vi "Main_Module.vi"(0 "Instances":string(tree)="Addition_8", 11 "Error_In":errorcluster) -> (15 "Error_Out":errorcluster)   [LabVIEW 2021]
doc: "This is the main module that performs the calculator operation"
uses:
  Controls/Queue_Operation_Select.ctl
  Drivers/QD_Main.vi
  Controls/State_and_Data.ctl
  Classes/Calculator/Calculator.lvclass
  <vilib>/Utility/miscctls.llb/LVMapReplaceAction.ctl
  Controls/Object_Data.ctl
  Controls/Object_and_instance.ctl
  Controls/INI_Operation_Select.ctl
  Controls/Main_Module_Data.ctl
  Drivers/QD_Calci.vi
panel:
  in  "Load":bool
  in  "Save":bool
  in  "Delete":bool
  in  "Add":bool
  in  "Math_Functions":T1(ring) caption="Math Functions"
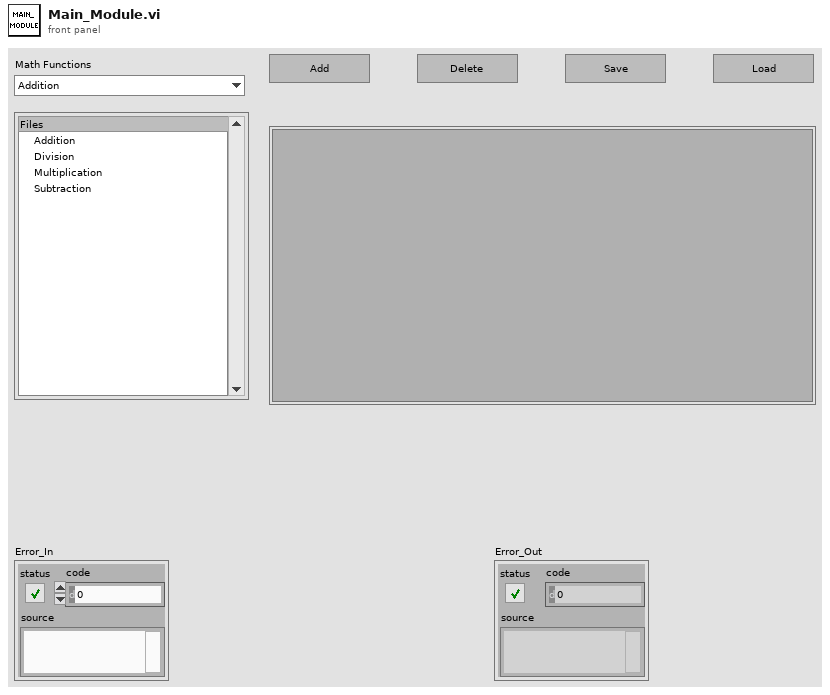
[diagram p1: front panel]
types:
  T1 = enum32{"Addition", "Division", "Multiplication", "Subtraction"}
  T2 = typedef "Queue_Operation_Select.ctl" = enum16{"Obtain_Queue", "Enqueue", "Enqueue_First", "Enqueue_N", "Lossy_Enqueue", "Preview", "Queue_Status", "Dequeue", "Flush", "Release_Queue"}
  T3 = typedef "Main_Module_Data.ctl" = cluster{"File_hierarchy_Reference":refnum<vi>, "Math_Function_Selected":string, "State_and_Data":T4, "Math_Functions":enum16{"Addition", "Division", "Multiplication", "Subtraction"}, "Parent_Class_Path":path, "Calculator.lvclass":refnum<class "Calculator.lvclass">, "Object_Data":T5, "Selected_Tag":string, "Calculator_File_Path":path, "Loaded_VI_Reference":refnum<vi>, "Loaded_Math_Function":string, "Loaded_Tag":string, "Total_Classes":string[], "INI_File_Path":path}
  T4 = typedef "State_and_Data.ctl" = cluster{"State":string, "Data":variant}
  T5 = typedef "Object_Data.ctl" = map{string, map{string, refnum<class "Calculator.lvclass">}}
  T6 = enum16{"Addition", "Division", "Multiplication", "Subtraction"}
  T7 = typedef "Object_and_instance.ctl" = cluster{"Object":refnum<class "Calculator.lvclass">, "Instance":string}
  T8 = typedef "INI_Operation_Select.ctl" = enum16{"Initialize", "Read", "Read_Key", "Write"}
  T9 = typedef "LVMapReplaceAction.ctl" = enum32{"Modify Entry only if found", "Add or Modify Entry", "Delete Entry"}
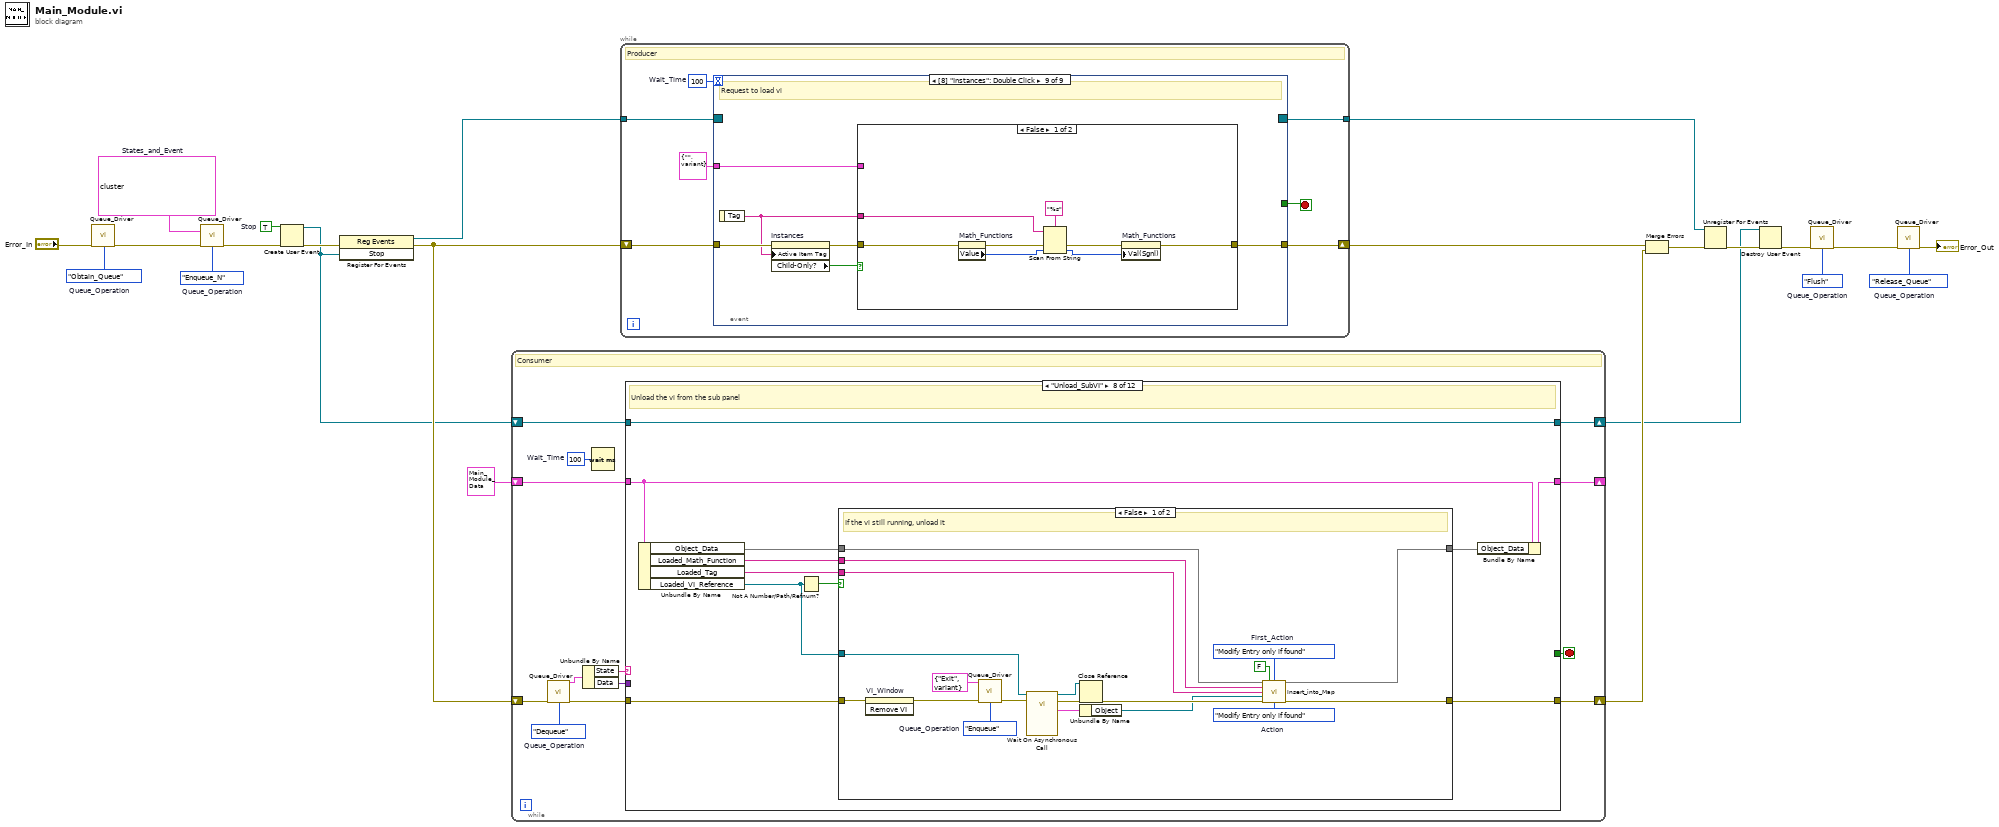
[diagram p0: block diagram]
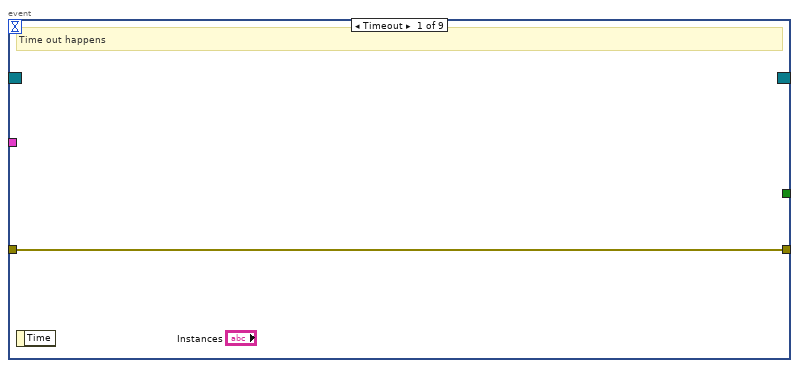
[diagram p2: hidden frame]
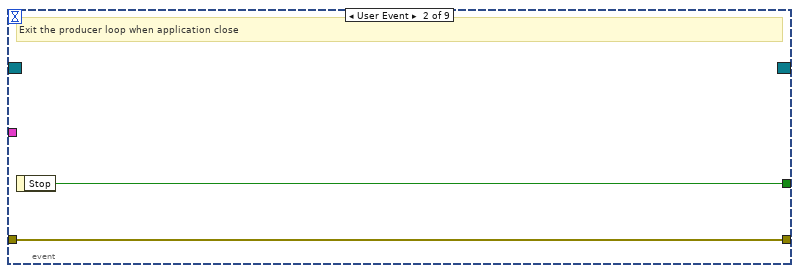
[diagram p3: hidden frame]
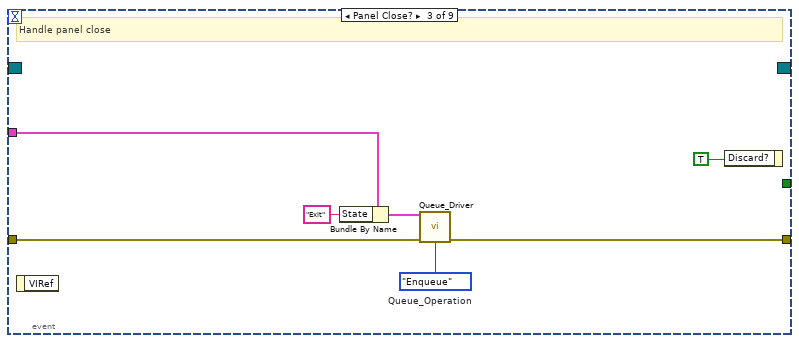
[diagram p4: hidden frame]
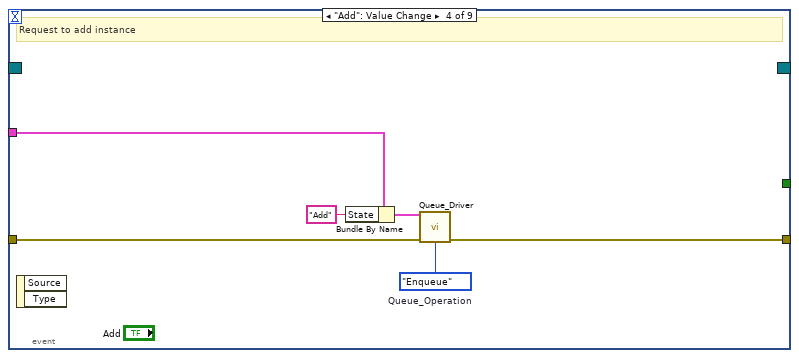
[diagram p5: hidden frame]
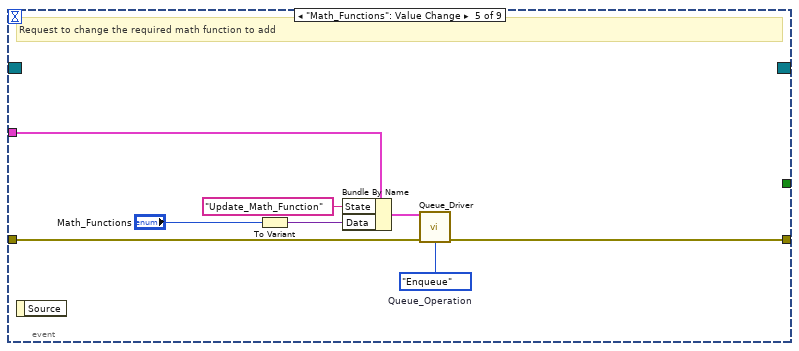
[diagram p6: hidden frame]
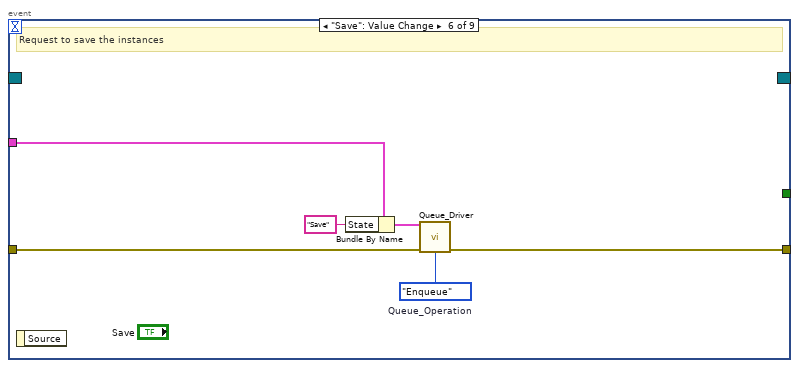
[diagram p7: hidden frame]
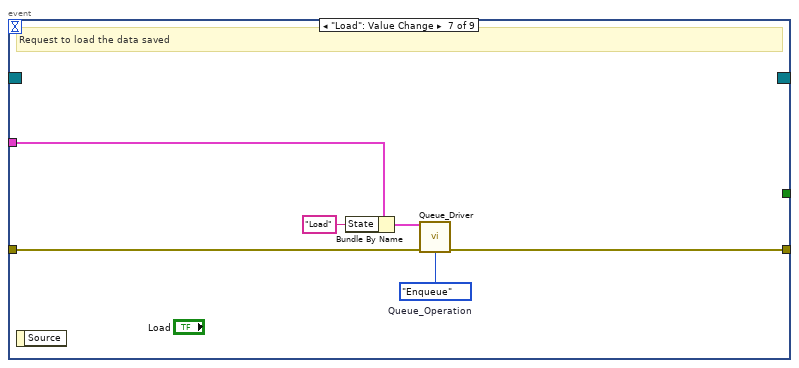
[diagram p8: hidden frame]
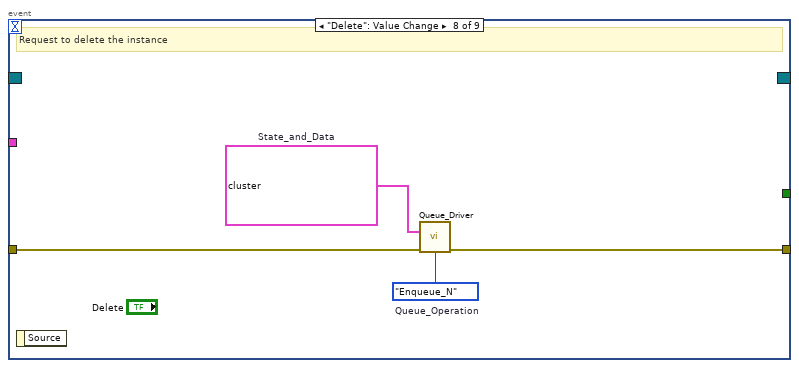
[diagram p9: hidden frame]
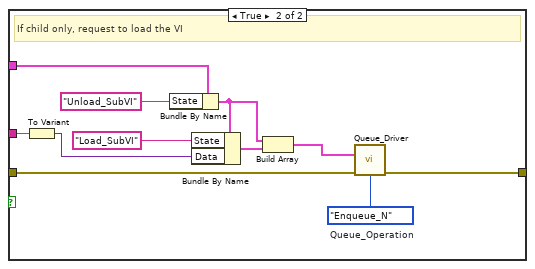
[diagram p10: hidden frame]
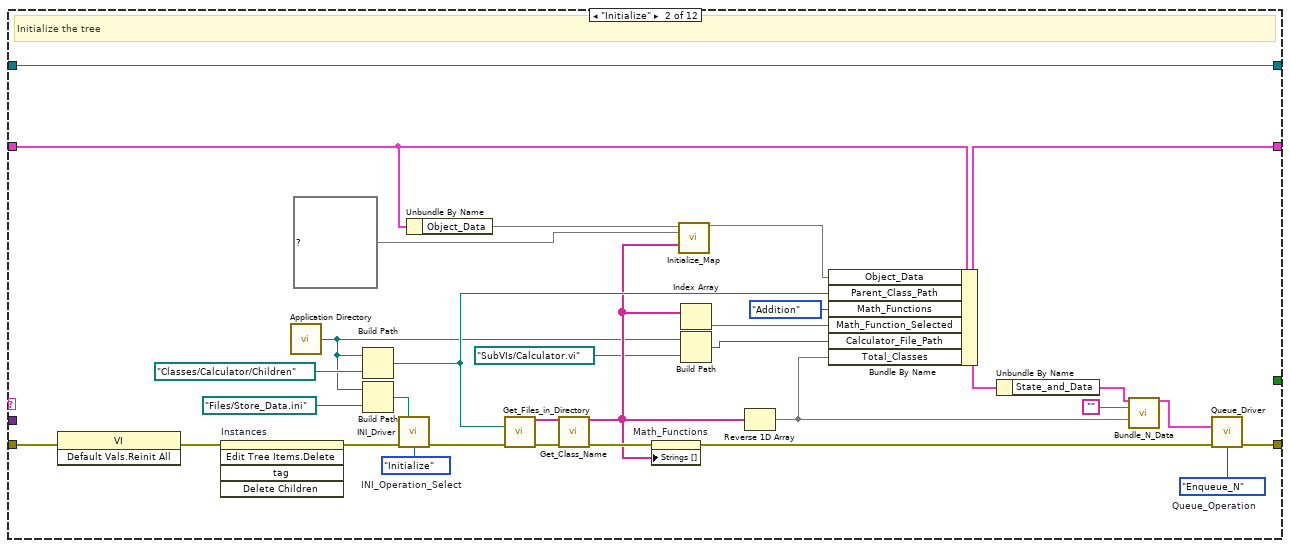
[diagram p12: hidden frame]
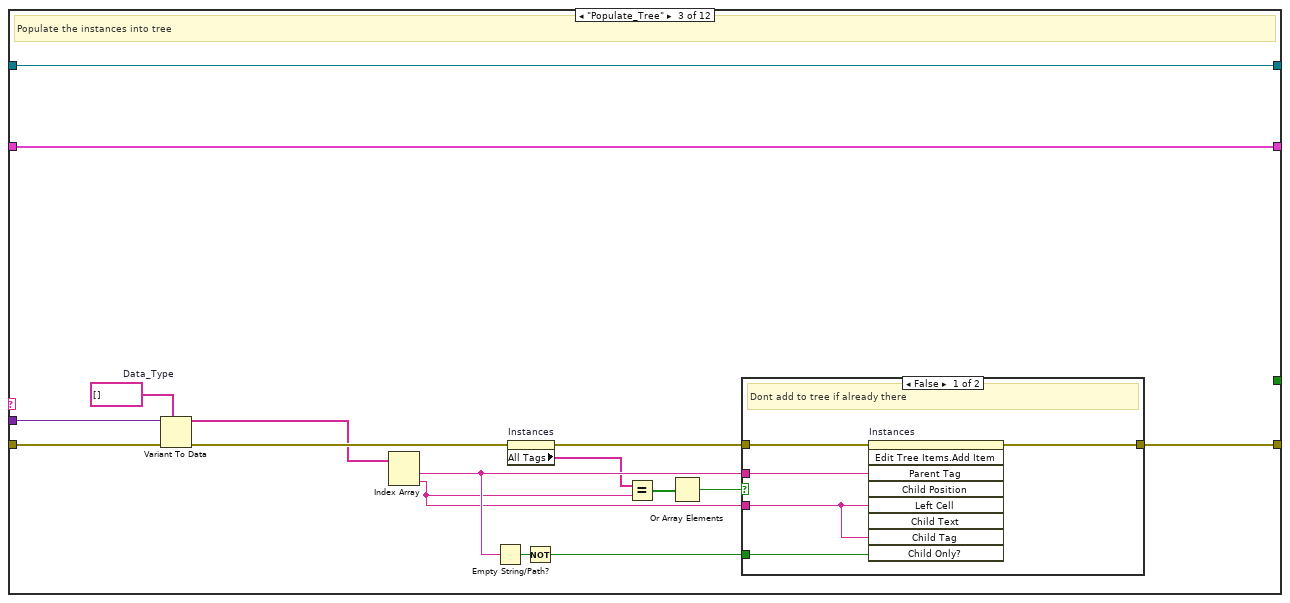
[diagram p13: hidden frame]
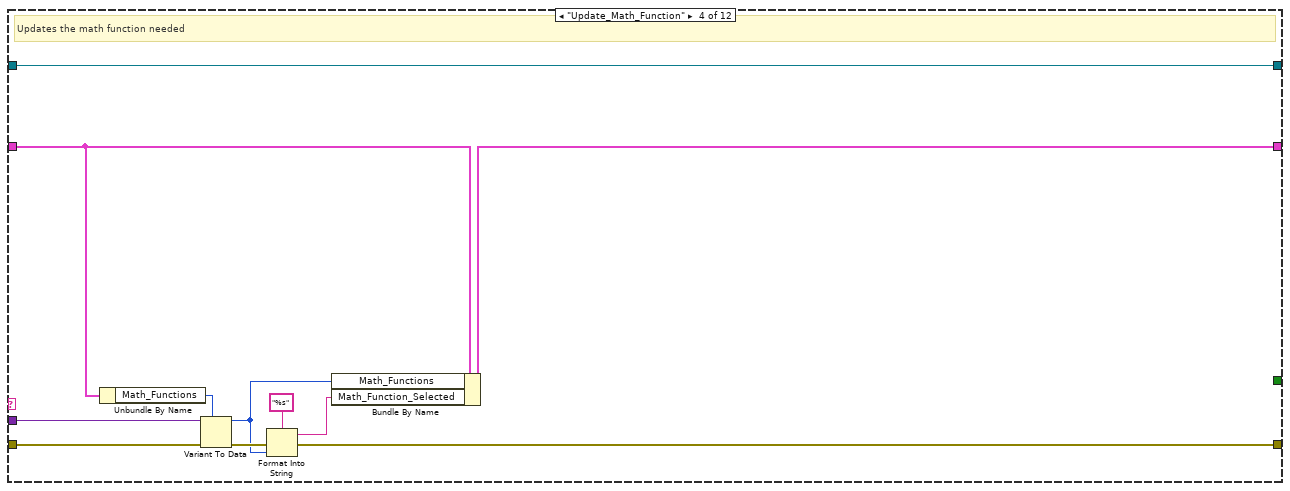
[diagram p15: hidden frame]
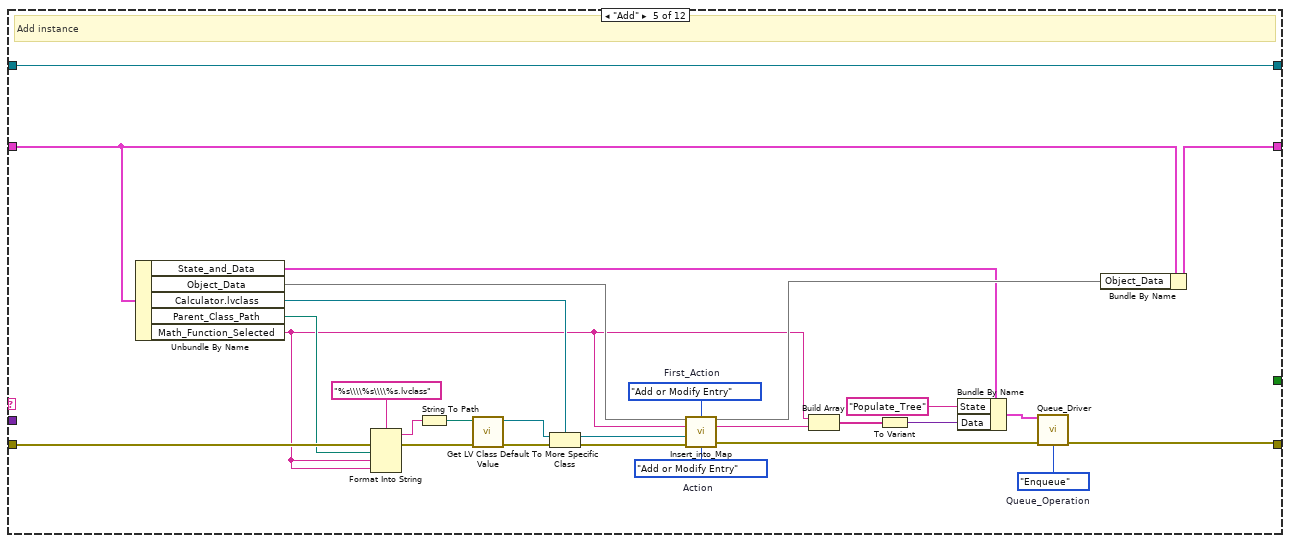
[diagram p16: hidden frame]
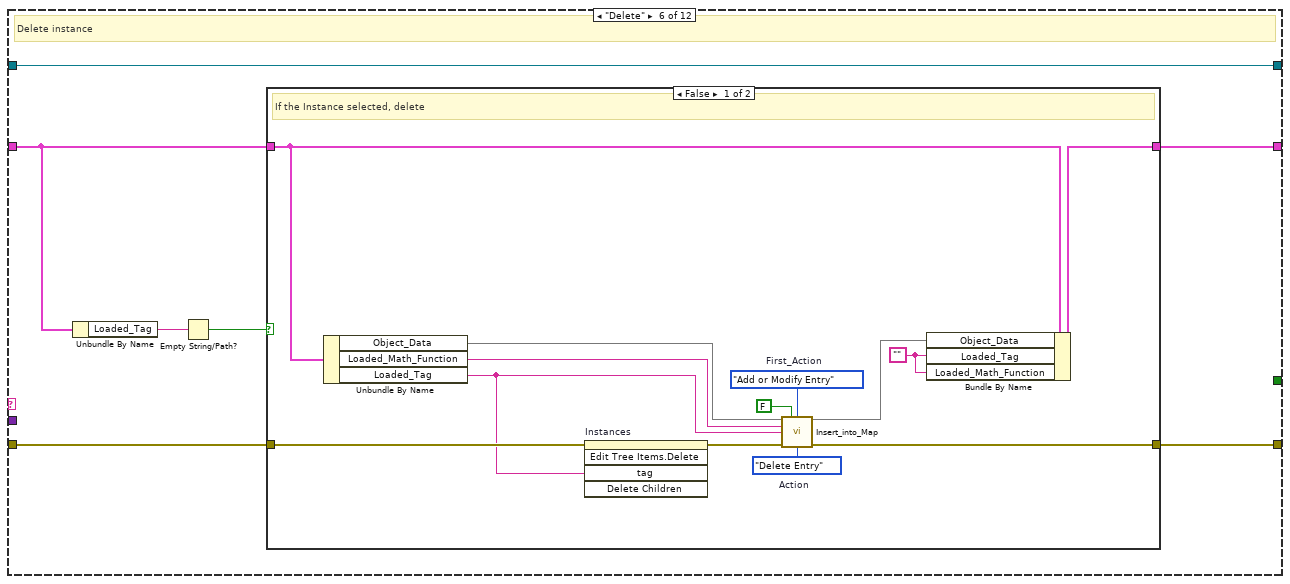
[diagram p17: hidden frame]
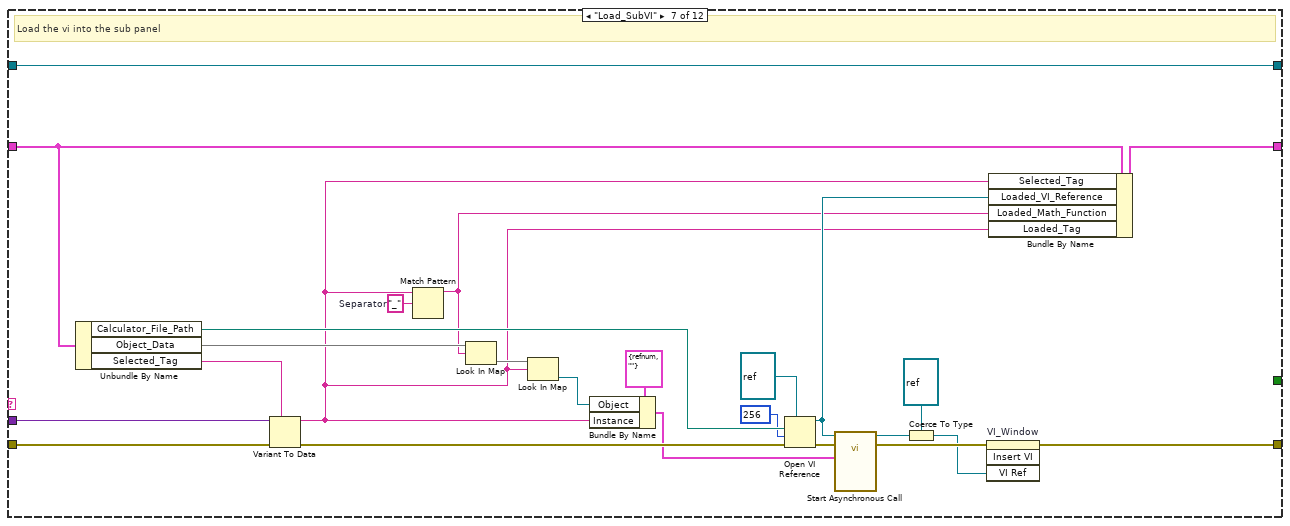
[diagram p19: hidden frame]
diagram:
  w4 = Queue_Operation_Select."Release_Queue"  # Queue_Operation
  w5 = Queue_Operation_Select."Flush"  # Queue_Operation
  w17 = TRUE  # Stop
  w1 = T4[] [{"State"="Initialize", "Data"=variant}, {"State"="Load", "Data"=variant}]  # States_and_Event
  w20 = Queue_Operation_Select."Enqueue_N"  # Queue_Operation
  w21 = Queue_Operation_Select."Obtain_Queue"  # Queue_Operation
  n1 = call-poly "Queue_Driver.vi"("Error_In"="Error_In", "Queue_Operation"=w21) -> ("Error_Out"=w22:errorcluster)  [unwired: 11 in, 2 out]
  n2 = call-poly "Queue_Driver.vi"("State_and_Data_N_In"=w1, "Error_In"=w22, "Queue_Operation"=w20) -> ("Error_Out"=w3:errorcluster)  [unwired: 10 in, 2 out]
  n3 = Create User Event(user event datatype=w17, error in=w3) -> (user event=w9:refnum<user-event>, error out=w18:errorcluster)
  n4 = register-events(error in=w18, w9) -> (reference out=w15:refnum<event-registration>, error out=w16:errorcluster)  [unwired: 1 in]
  n5 = while {
    shift-right: [w28] -> w8
    shift-left: w9 -> [w29]
    shift-right: [w27] -> _
    shift-left: T3 {"File_hierarchy_Reference"=refnum, "Math_Function_Selected"="", "State_and_Data"={"State"="", "Data"=variant}, "Math_Functions"=enum."Addition", "Parent_Class_Path"=path "", "Calculator.lvclass"=refnum, "Object_Data"={}, "Selected_Tag"="", "Calculator_File_Path"=path "", "Loaded_VI_Reference"=refnum, "Loaded_Math_Function"="", "Loaded_Tag"="", "Total_Classes"=[], "INI_File_Path"=path ""} -> [w30]
    shift-right: [w26] -> w13
    shift-left: w16 -> [w36]
    stop <- w25 stop-if-true
    w24 = u32 100  # Wait_Time
    w34 = Queue_Operation_Select."Dequeue"  # Queue_Operation
    # "Consumer"
    n6 = call-poly "Queue_Driver.vi"("Error_In"=w36, "Queue_Operation"=w34) -> ("State_and_Data_Out"=w33:T4, "Error_Out"=w35:errorcluster)  [unwired: 11 in, 1 out]
    n7 = Unbundle By Name(w33) -> ("State"=w32:string, "Data"=w31:variant)
    n8 = Wait (ms)(milliseconds to wait=w24) -> ()  [unwired: 1 out]
    n9 = case shown="\"Unload_SubVI\"" w32 {
      tunnel: [w39 w62 w83 w96 w113 w136 w176 w186 w212 w249 w255 w265] -> w26
      tunnel: w35 -> [w39 w70 w86 w103 w131 w138 w178 w181 w211 w250 w259 w267]
      tunnel: w31 -> [_ _ w81 w100 _ _ w177 _ _ _ w260 _]
      tunnel: w30 -> [w38 w52 w85 w98 w129 w134 w173 w188 w218 w245 w256 w266]
      tunnel: [w38 w42 w85 w97 w120 w135 w172 w187 w215 w245 w256 w266] -> w27
      tunnel: w29 -> [w37 w69 w84 w102 w130 w137 w174 w189 w225 w251 w261 w264]
      tunnel: [w37 w69 w84 w102 w130 w137 w174 w189 w225 w251 w261 w263] -> w28
      tunnel: [_ _ _ _ _ _ _ _ _ _ _ w262] -> w25
      frame Default {
      }
      frame "Initialize" {
        w45 = INI_Operation_Select."Initialize"  # INI_Operation_Select
        w61 = Queue_Operation_Select."Enqueue_N"  # Queue_Operation
        # "Initialize the tree"
        n10 = invoke class="VI" method="Default Vals.Reinit All"(error in=w70) -> (error out=w40:errorcluster)  [unwired: 2 in, 2 out]
        n11 = invoke on="Instances" class="Tree (strict)" method="Edit Tree Items.Delete"(error in=w40) -> (error out=w67:errorcluster)  [unwired: 4 in, 4 out]
        n12 = call <vilib>:"Application Directory.vi"() -> ("Application Directory"=w43:path)
        n13 = Build Path(base path=w43, name or relative path=path "Classes/Calculator/Children") -> (appended path=w58:path)
        n14 = Build Path(base path=w43, name or relative path=path "Files/Store_Data.ini") -> (appended path=w44:path)
        n15 = call "INI_Driver.vi"("Config_File_Path"=w44, "Error_Out"=w67, "INI_Operation_Select"=w45) -> ("Error_Out"=w46:errorcluster)  [unwired: 10 in, 2 out]
        n16 = Unbundle By Name(w52) -> ("Object_Data"=w51:T5)
        n17 = call "Get_Files_in_Directory.vi"("File_Path"=w58, "Error_In"=w46) -> ("File_Names_Out"=w64:string[], "Error_Out"=w66:errorcluster)  [unwired: 12 in]
        n18 = call "Get_Class_Name.vi"("File_Names"=w64, "Error_In"=w66) -> ("Class_Names"=w55:string[], "Error_Out"=w65:errorcluster)  [unwired: 12 in]
        n19 = property on="Math_Functions" class="Enum (strict)"(error in=w65, "Strings []"=w55) -> (error out=w63:errorcluster)  [unwired: 1 in, 1 out]
        n20 = call "Initialize_Map.vi"("Object_Data_In"=w51, "Default_Data"=map{string, refnum<class "Calculator.lvclass">} {} ("Object_Data"), "Class_Names"=w55) -> ("Object_Data_Out"=w53:T5)  [unwired: 12 in]
        n21 = Index Array(array=w55) -> (element=w56:string)  [unwired: 1 in]
        n22 = Build Path(base path=w43, name or relative path=path "SubVIs/Calculator.vi") -> (appended path=w49:path)
        n23 = Reverse 1D Array(array=w55) -> (reversed array=w48:string[])
        n24 = Bundle By Name(cluster=w52, "Object_Data"=w53, "Parent_Class_Path"=w58, "Math_Functions"=T6."Addition", "Math_Function_Selected"=w56, "Calculator_File_Path"=w49, "Total_Classes"=w48) -> (w42:T3)
        n25 = Unbundle By Name(w42) -> ("State_and_Data"=w41:T4)
        n26 = call "Bundle_N_Data.vi"("Data_Type"=w41, "Parent"="", "Children_Names"=w48) -> ("Data_Out"=w59:T4[])  [unwired: 12 in]
        n27 = call-poly "Queue_Driver.vi"("State_and_Data_N_In"=w59, "Error_In"=w63, "Queue_Operation"=w61) -> ("Error_Out"=w62:errorcluster)  [unwired: 10 in, 2 out]
      }
      frame "Populate_Tree" {
        w80 = string[] []  # Data_Type
        # "Populate the instances into tree"
        n28 = Variant To Data(error in=w86, type=w80, Variant=w81) -> (data=w79:string[], error out=w82:errorcluster)
        n29 = Index Array(array=w79) -> (element #1=w78:string, element #2=w73:string)  [unwired: 2 in]
        n30 = Empty String/Path?(string/path=w78) -> (empty?=w77:bool)
        n31 = property on="Instances" class="Tree (strict)"(error in=w82) -> (error out=w75:errorcluster, "All Tags"=w74:string[])  [unwired: 1 in, 1 out]
        n32 = Not(x=w77) -> (.not. x?=w76:bool)
        n33 = Equal?(x=w74, y=w73) -> (x = y?=w72:bool[])
        n34 = Or Array Elements(Boolean array=w72) -> (logical OR=w71:bool)
        n35 = case shown="False" w71 {
          tunnel: [w91 w92] -> w83
          tunnel: w78 -> [w90 _]
          tunnel: w76 -> [w89 _]
          tunnel: w75 -> [w88 w92]
          tunnel: w73 -> [w87 _]
          frame False {
            # "Dont add to tree if already there"
            n36 = invoke on="Instances" class="Tree (strict)" method="Edit Tree Items.Add Item"(error in=w88, "Parent Tag"=w90, "Left Cell"=w87, "Child Tag"=w87, "Child Only?"=w89) -> (error out=w91:errorcluster)  [unwired: 4 in, 8 out]
          }
          frame True {
          }
        }
      }
      frame "Update_Math_Function" {
        # "Updates the math function needed"
        n37 = Unbundle By Name(w98) -> ("Math_Functions"=w99:T6)
        n38 = Variant To Data(error in=w103, type=w99, Variant=w100) -> (data=w93:T6, error out=w101:errorcluster)
        n39 = Format Into String(format string="%s", error in=w101, w93) -> (resulting string=w94:string, error out=w96:errorcluster)  [unwired: 1 in]
        n40 = Bundle By Name(cluster=w98, "Math_Functions"=w93, "Math_Function_Selected"=w94) -> (w97:T3)
      }
      frame "Add" {
        w105 = LVMapReplaceAction."Add or Modify Entry"  # First_Action
        w108 = LVMapReplaceAction."Add or Modify Entry"  # Action
        w115 = Queue_Operation_Select."Enqueue"  # Queue_Operation
        # "Add instance"
        n41 = Unbundle By Name(w129) -> ("State_and_Data"=w104:T4, "Object_Data"=w119:T5, "Calculator.lvclass"=w122:refnum<class "Calculator.lvclass">, "Parent_Class_Path"=w127:path, "Math_Function_Selected"=w109:string)
        n42 = Format Into String(format string="%s\\\\%s\\\\%s.lvclass", error in=w131, w127, w109, w109) -> (resulting string=w126:string, error out=w125:errorcluster)  [unwired: 1 in]
        n43 = String To Path(string=w126) -> (path=w124:path)
        n44 = call <vilib>:"Get LV Class Default Value.vi"("error in (no error)"=w125, "class path"=w124) -> ("error out"=w121:errorcluster, "object"=w123:refnum<class>)  [unwired: 8 in]
        n45 = To More Specific Class(target class=w122, reference=w123, error in=w121) -> (specific class reference=w106:refnum<class "Calculator.lvclass">, error out=w107:errorcluster)
        n46 = call "Insert_into_Map.vi"("Object_Data_In"=w119, "First_Action"=w105, "First_Key"=w109, "Calculator.lvclass"=w106, "Error_In"=w107, "Second_Action"=w108) -> ("Object_Data_Out"=w118:T5, "Second_Key"=w112:string, "error out"=w114:errorcluster)  [unwired: 7 in]
        n47 = Build Array(w109, w112) -> (w110:string[])
        n48 = To Variant(anything=w110) -> (Variant=w111:variant)
        n49 = Bundle By Name(cluster=w104, "State"="Populate_Tree", "Data"=w111) -> (w117:T4)
        n50 = call-poly "Queue_Driver.vi"("State_and_Data_In"=w117, "Error_In"=w114, "Queue_Operation"=w115) -> ("Error_Out"=w113:errorcluster)  [unwired: 10 in, 2 out]
        n51 = Bundle By Name(cluster=w129, "Object_Data"=w118) -> (w120:T3)
      }
      frame "Delete" {
        # "Delete instance"
        n52 = Unbundle By Name(w134) -> ("Loaded_Tag"=w133:string)
        n53 = Empty String/Path?(string/path=w133) -> (empty?=w132:bool)
        n54 = case shown="False" w132 {
          tunnel: w138 -> [w151 w153]
          tunnel: w134 -> [w150 w152]
          tunnel: [w148 w153] -> w136
          tunnel: [w144 w152] -> w135
          frame False {
            w140 = LVMapReplaceAction."Add or Modify Entry"  # First_Action
            w142 = ""
            w141 = LVMapReplaceAction."Delete Entry"  # Action
            # "If the Instance selected, delete"
            n55 = Unbundle By Name(w150) -> ("Object_Data"=w147:T5, "Loaded_Math_Function"=w146:string, "Loaded_Tag"=w145:string)
            n56 = invoke on="Instances" class="Tree (strict)" method="Edit Tree Items.Delete"(error in=w151, "tag"=w145) -> (error out=w149:errorcluster)  [unwired: 3 in, 4 out]
            n57 = call "Insert_into_Map.vi"("Object_Data_In"=w147, "Create_Second_Key (T)"=FALSE, "First_Action"=w140, "First_Key"=w146, "Second_Key"=w145, "Error_In"=w149, "Second_Action"=w141) -> ("Object_Data_Out"=w143:T5, "error out"=w148:errorcluster)  [unwired: 6 in, 1 out]
            n58 = Bundle By Name(cluster=w150, "Object_Data"=w143, "Loaded_Tag"=w142, "Loaded_Math_Function"=w142) -> (w144:T3)
          }
          frame True {
          }
        }
      }
      frame "Load_SubVI" {
        w159 = "_"  # Separator
        # "Load the vi into the sub panel"
        n59 = Unbundle By Name(w173) -> ("Calculator_File_Path"=w166:path, "Object_Data"=w168:T5, "Selected_Tag"=w175:string)
        n60 = Variant To Data(error in=w178, type=w175, Variant=w177) -> (data=w154:string, error out=w160:errorcluster)
        n61 = Match Pattern(string=w154, regular expression=w159) -> (before substring=w158:string)  [unwired: 1 in, 3 out]
        n62 = Look In Map(map=w168, key=w158) -> (value=w167:map{string, refnum<class "Calculator.lvclass">})  [unwired: 1 in, 1 out]
        n63 = Look In Map(map=w167, key=w154) -> (value=w155:refnum<class "Calculator.lvclass">)  [unwired: 1 in, 1 out]
        n64 = Bundle By Name(cluster=T7 {"Object"=refnum, "Instance"=""}, "Object"=w155, "Instance"=w154) -> (w156:T7)
        n65 = Open VI Reference(type specifier VI Refnum (for type only)=refnum<vi> refnum, vi path=w166, options=256, error in (no error)=w160) -> (vi reference=w161:refnum<vi>, error out=w171:errorcluster)  [unwired: 2 in]
        n66 = call-by-ref "Start Asynchronous Call"(reference=w161, error in=w171, "Object_and_Instance_In"=w156) -> (reference out=w165:refnum<vi>, error out=w170:errorcluster)  [unwired: 12 in, 3 out]
        n67 = Coerce To Type(0:w165, 1:refnum<vi> refnum ("This VI")) -> (2:w162:refnum<vi>)
        n68 = invoke on="VI_Window" class="SubPnl" method="Insert VI"(error in=w170, "VI Ref"=w162) -> (error out=w176:errorcluster)  [unwired: 2 in, 3 out]
        n69 = Bundle By Name(cluster=w173, "Selected_Tag"=w154, "Loaded_VI_Reference"=w161, "Loaded_Math_Function"=w158, "Loaded_Tag"=w154) -> (w172:T3)
      }
      frame "Unload_SubVI" {
        # "Unload the vi from the sub panel"
        n70 = Unbundle By Name(w188) -> ("Object_Data"=w185:T5, "Loaded_Math_Function"=w184:string, "Loaded_Tag"=w183:string, "Loaded_VI_Reference"=w180:refnum<vi>)
        n71 = Not A Number/Path/Refnum?(number/path/refnum=w180) -> (NaN/Path/Refnum?=w179:bool)
        n72 = case shown="False" w179 {
          tunnel: w181 -> [w199 w209]
          tunnel: w180 -> [w207 _]
          tunnel: [w205 w209] -> w186
          tunnel: w185 -> [w204 w210]
          tunnel: w184 -> [w203 _]
          tunnel: w183 -> [w202 _]
          tunnel: [w200 w210] -> w182
          frame False {
            w190 = LVMapReplaceAction."Modify Entry only if found"  # First_Action
            w196 = Queue_Operation_Select."Enqueue"  # Queue_Operation
            w201 = LVMapReplaceAction."Modify Entry only if found"  # Action
            # "If the vi still running, unload it"
            n73 = invoke on="VI_Window" class="SubPnl" method="Remove VI"(error in=w199) -> (error out=w192:errorcluster)  [unwired: 2 in, 2 out]
            n74 = call-poly "Queue_Driver.vi"("State_and_Data_In"=T4 {"State"="Exit", "Data"=variant} ("State_and_Data"), "Error_In"=w192, "Queue_Operation"=w196) -> ("Error_Out"=w198:errorcluster)  [unwired: 10 in, 2 out]
            n75 = call-by-ref "Wait On Asynchronous Call"(reference=w207, error in=w198) -> (reference out=w206:refnum<vi>, error out=w208:errorcluster, "Object_and_instance_Out"=w194:T7)  [unwired: 13 in, 2 out]
            n76 = Close Reference(reference=w206, error in (no error)=w208) -> (error out=w195:errorcluster)
            n77 = Unbundle By Name(w194) -> ("Object"=w193:refnum<class "Calculator.lvclass">)
            n78 = call "Insert_into_Map.vi"("Object_Data_In"=w204, "Create_Second_Key (T)"=FALSE, "First_Action"=w190, "First_Key"=w203, "Second_Key"=w202, "Calculator.lvclass"=w193, "Error_In"=w195, "Second_Action"=w201) -> ("Object_Data_Out"=w200:T5, "error out"=w205:errorcluster)  [unwired: 5 in, 1 out]
          }
          frame True {
          }
        }
        n79 = Bundle By Name(cluster=w188, "Object_Data"=w182) -> (w187:T3)
      }
      frame "Load" {
        w221 = "Map"  # Key
        w222 = "Data"  # Section
        w223 = INI_Operation_Select."Read"  # INI_Operation_Select
        # "Load the saved instances"
        n80 = call "INI_Driver.vi"("Section"=w222, "Key"=w221, "Error_Out"=w211, "INI_Operation_Select"=w223) -> ("Data_Out"=w219:string, "Error_Out"=w224:errorcluster)  [unwired: 9 in, 1 out]
        n81 = Unbundle By Name(w218) -> ("Total_Classes"=w213:string[], "Object_Data"=w217:T5)
        n82 = Unflatten From XML(xml string=w219, type=w217, error in (no error)=w224) -> (value=w214:T5, error out=w220:errorcluster)
        n83 = for {
          tunnel: w214 -> [w229]
          tunnel: w213 -> [w227] mode=indexing
          tunnel: w220 -> [w231]
          tunnel: [w226] -> w216 mode=indexing
          # "Send the instance to populate the tree"
          n84 = Look In Map(map=w229, key=w227) -> (value=w228:map{string, refnum<class "Calculator.lvclass">})  [unwired: 1 in, 1 out]
          n85 = for {
            tunnel: w228 -> [w240] mode=indexing
            tunnel: w227 -> [w234]
            tunnel: w231 -> [w232]
            tunnel: [w242] -> w230 mode=indexing
            w241 = Queue_Operation_Select."Enqueue"  # Queue_Operation
            n86 = Unbundle(w240) -> (w233:string)  [unwired: 1 out]
            n87 = Build Array(w234, w233) -> (w235:string[])
            n88 = To Variant(anything=w235) -> (Variant=w237:variant)
            n89 = Bundle By Name(cluster=T4 {"State"="", "Data"=variant} ("State_and_Data"), "State"="Populate_Tree", "Data"=w237) -> (w238:T4)
            n90 = call-poly "Queue_Driver.vi"("State_and_Data_In"=w238, "Error_In"=w232, "Queue_Operation"=w241) -> ("Error_Out"=w242:errorcluster)  [unwired: 10 in, 2 out]
          }
          n91 = Merge Errors(w230) -> (w226:errorcluster)
        }
        n92 = Bundle By Name(cluster=w218, "Object_Data"=w214) -> (w215:T3)
        n93 = Merge Errors(w216) -> (w212:errorcluster)
      }
      frame "Save" {
        w246 = "Map"  # Key
        w247 = "Data"  # Section
        w248 = INI_Operation_Select."Write"  # INI_Operation_Select
        # "Save the instances"
        n94 = Unbundle By Name(w245) -> ("Object_Data"=w244:T5)
        n95 = Flatten To XML(6:w244) -> (2:w243:string)
        n96 = call "INI_Driver.vi"("Data_In"=w243, "Section"=w247, "Key"=w246, "Error_Out"=w250, "INI_Operation_Select"=w248) -> ("Error_Out"=w249:errorcluster)  [unwired: 8 in, 2 out]
      }
      frame "Error" {
        w254 = Queue_Operation_Select."Enqueue"  # Queue_Operation
        # "Handle error"
        n97 = Variant To Data(error in=w259, type=w259, Variant=w260) -> (data=w253:errorcluster, error out=w258:errorcluster)
        n98 = call "Analyse_Error.vi"("Error_Under_Analysis"=w253, "Error_In"=w258) -> ("State_and_Data"=w252:T4, "Error_Out"=w257:errorcluster)  [unwired: 12 in]
        n99 = call-poly "Queue_Driver.vi"("State_and_Data_In"=w252, "Error_In"=w257, "Queue_Operation"=w254) -> ("Error_Out"=w255:errorcluster)  [unwired: 10 in, 2 out]
      }
      frame "Exit" {
        # "Exit the application"
        n100 = disable-structure shown="RUN_TIME_ENGINE==True" {
          disable-tunnel: [w268 w272] -> w262
          frame condition #0 {
            w268 = TRUE  # Stop
            # "Run time mode"
          }
          frame condition #1 (active) {
            w269 = "No"  # Cont
            w270 = "Yes"  # Stop
            w271 = "Do you want to stop execution"  # Message
            # "Developer mode"
            n101 = Two Button Dialog(message=w271, 1:w269, 2:w270) -> (T button?=w272:bool)
          }
        }
        n102 = Generate User Event(user event=w264, event data cluster=w262, error in=w267) -> (user event out=w263:refnum<user-event>, error out=w265:errorcluster)  [unwired: 1 in]
      }
    }
  }
  n103 = while {
    tunnel: w15 -> [w278]
    shift-right: [w276] -> w14
    shift-left: w16 -> [w279]
    tunnel: [w274] -> w11
    stop <- w277 stop-if-true
    w275 = 100  # Wait_Time
    # "Producer"
    n104 = event shown="[8] \"Instances\": Double Click" {
      selector: w278 -> [_ _ _ _ _ _ _ _ _]
      dyn-events: [_ _ _ _ _ _ _ _ _] -> w274
      timeout: w275 -> [_ _ _ _ _ _ _ _ _]
      tunnel: w279 -> [w280 w282 w286 w293 w301 w307 w313 w318 w324]
      tunnel: [w280 w282 w285 w292 w300 w306 w312 w317 w325] -> w276
      tunnel: [_ w281 _ _ _ _ _ _ _] -> w277
      tunnel: T4 {"State"="", "Data"=variant} ("State_and_Data") -> [_ _ w283 w290 w296 w304 w310 _ w320]
      event Timeout {
        # "Time out happens"
        n105 = event-data() -> ()  [unwired: 1 in, 1 out]
      }
      event User Event {
        # "Exit the producer loop when application close"
        n106 = event-data() -> ("Stop"=w281:bool)  [unwired: 1 in]
      }
      event Panel Close? {
        w287 = Queue_Operation_Select."Enqueue"  # Queue_Operation
        # "Handle panel close"
        n107 = event-data() -> ()  [unwired: 1 in, 1 out]
        n108 = Bundle By Name(cluster=w283, "State"="Exit") -> (w284:T4)
        n109 = call-poly "Queue_Driver.vi"("State_and_Data_In"=w284, "Error_In"=w286, "Queue_Operation"=w287) -> ("Error_Out"=w285:errorcluster)  [unwired: 10 in, 2 out]
        n110 = event-data("Discard?"=TRUE) -> ()  [unwired: 1 in, 1 out]
      }
      event "Add": Value Change {
        w294 = Queue_Operation_Select."Enqueue"  # Queue_Operation
        # "Request to add instance"
        n111 = event-data() -> ()  [unwired: 1 in, 2 out]
        n112 = Bundle By Name(cluster=w290, "State"="Add") -> (w291:T4)
        n113 = call-poly "Queue_Driver.vi"("State_and_Data_In"=w291, "Error_In"=w293, "Queue_Operation"=w294) -> ("Error_Out"=w292:errorcluster)  [unwired: 10 in, 2 out]
      }
      event "Math_Functions": Value Change {
        w302 = Queue_Operation_Select."Enqueue"  # Queue_Operation
        # "Request to change the required math function to add"
        n114 = event-data() -> ()  [unwired: 1 in, 1 out]
        n115 = To Variant(anything="Math_Functions") -> (Variant=w297:variant)
        n116 = Bundle By Name(cluster=w296, "State"="Update_Math_Function", "Data"=w297) -> (w299:T4)
        n117 = call-poly "Queue_Driver.vi"("State_and_Data_In"=w299, "Error_In"=w301, "Queue_Operation"=w302) -> ("Error_Out"=w300:errorcluster)  [unwired: 10 in, 2 out]
      }
      event "Save": Value Change {
        w308 = Queue_Operation_Select."Enqueue"  # Queue_Operation
        # "Request to save the instances"
        n118 = event-data() -> ()  [unwired: 1 in, 1 out]
        n119 = Bundle By Name(cluster=w304, "State"="Save") -> (w305:T4)
        n120 = call-poly "Queue_Driver.vi"("State_and_Data_In"=w305, "Error_In"=w307, "Queue_Operation"=w308) -> ("Error_Out"=w306:errorcluster)  [unwired: 10 in, 2 out]
      }
      event "Load": Value Change {
        w314 = Queue_Operation_Select."Enqueue"  # Queue_Operation
        # "Request to load the data saved"
        n121 = event-data() -> ()  [unwired: 1 in, 1 out]
        n122 = Bundle By Name(cluster=w310, "State"="Load") -> (w311:T4)
        n123 = call-poly "Queue_Driver.vi"("State_and_Data_In"=w311, "Error_In"=w313, "Queue_Operation"=w314) -> ("Error_Out"=w312:errorcluster)  [unwired: 10 in, 2 out]
      }
      event "Delete": Value Change {
        w319 = Queue_Operation_Select."Enqueue_N"  # Queue_Operation
        w316 = T4[] [{"State"="Unload_SubVI", "Data"=variant}, {"State"="Delete", "Data"=variant}]  # State_and_Data
        # "Request to delete the instance"
        n124 = event-data() -> ()  [unwired: 1 in, 1 out]
        n125 = call-poly "Queue_Driver.vi"("State_and_Data_N_In"=w316, "Error_In"=w318, "Queue_Operation"=w319) -> ("Error_Out"=w317:errorcluster)  [unwired: 10 in, 2 out]
      }
      event "Instances": Double Click {
        # "Request to load vi"
        n126 = event-data() -> ("Tag"=w322:string)  [unwired: 1 in]
        n127 = property on="Instances" class="Tree (strict)"(error in=w324, "Active Item Tag"=w322) -> (error out=w323:errorcluster, "Child-Only?"=w321:bool)  [unwired: 1 in, 1 out]
        n128 = case shown="False" w321 {
          tunnel: [w333 w344] -> w325
          tunnel: w323 -> [w327 w340]
          tunnel: w322 -> [w331 w339]
          tunnel: w320 -> [_ w334]
          frame False {
            n129 = property on="Math_Functions" class="Enum (strict)"(error in=w327) -> (error out=w328:errorcluster, "Value"=w326:T1)  [unwired: 1 in, 1 out]
            n130 = Scan From String(format string="%s", input string=w331, error in=w328, default 1=w326) -> (error out=w332:errorcluster, output 1=w329:T1)  [unwired: 1 in, 2 out]
            n131 = property on="Math_Functions" class="Enum (strict)"(error in=w332, "Val(Sgnl)"=w329) -> (error out=w333:errorcluster)  [unwired: 1 in, 1 out]
          }
          frame True {
            w341 = Queue_Operation_Select."Enqueue_N"  # Queue_Operation
            # "If child only, request to load the VI"
            n132 = To Variant(anything=w339) -> (Variant=w342:variant)
            n133 = Bundle By Name(cluster=w334, "State"="Unload_SubVI") -> (w337:T4)
            n134 = Bundle By Name(cluster=w337, "State"="Load_SubVI", "Data"=w342) -> (w338:T4)
            n135 = Build Array(w337, w338) -> (w336:T4[])
            n136 = call-poly "Queue_Driver.vi"("State_and_Data_N_In"=w336, "Error_In"=w340, "Queue_Operation"=w341) -> ("Error_Out"=w344:errorcluster)  [unwired: 10 in, 2 out]
          }
        }
      }
    }
  }
  n137 = Merge Errors(w14, w13) -> (w12:errorcluster)
  n138 = Unregister For Events(event registration refnum=w11, error in=w12) -> (error out=w10:errorcluster)
  n139 = Destroy User Event(user event=w8, error in=w10) -> (error out=w7:errorcluster)
  n140 = call-poly "Queue_Driver.vi"("Error_In"=w7, "Queue_Operation"=w5) -> ("Error_Out"=w6:errorcluster)  [unwired: 11 in, 2 out]
  n141 = call-poly "Queue_Driver.vi"("Error_In"=w6, "Queue_Operation"=w4) -> ("Error_Out"=→"Error_Out":errorcluster)  [unwired: 11 in, 2 out]
